vi "magazine_periodic.vi"(9 "Reverse":bool, 10 "Outtake":bool, 11 "Intake":bool) -> (2 "Stator Current":dbl)   [LabVIEW 2020]
uses:
  <vilib>/Rock Robotics/WPI/ThirdParty/Phoenix-LabVIEW/Motor Controller/Controls/CTRE_Phoenix_MotorControl_StatorCurrentLimitConfiguration.ctl
  <vilib>/Rock Robotics/WPI/ThirdParty/Phoenix-LabVIEW/Motor Controller/Controls/CTRE_Phoenix_MotorControl_ControlMode.ctl
  TitanLib/Lib/Piston Hold.vi
  <vilib>/Rock Robotics/WPI/Solenoid/WPI_SolenoidSetEnum.vi
  <vilib>/Rock Robotics/WPI/ThirdParty/Phoenix-LabVIEW/Motor Controller/Get/CTRE_Phoenix_MotorController_GetSupplyAndStatorCurrent_Enhanced.vi
  TitanLib/Lib/TitanLib.lvlib
panel:
  in  "Input":bool
  in  "Stator Current Limit Configuration":T1
  out "Sensor Values":cluster{i16, i16}(graph)
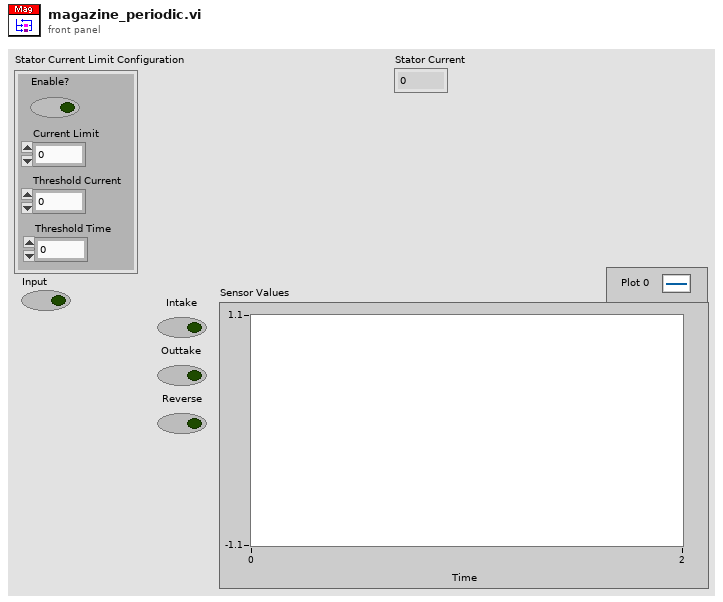
[diagram p1: front panel]
types:
  T1 = typedef "CTRE_Phoenix_MotorControl_StatorCurrentLimitConfiguration.ctl" = cluster{"Enable?":bool, "Current Limit":dbl, "Threshold Current":dbl, "Threshold Time":dbl}
  T2 = typedef "WPI_DigitalInputDevRef.ctl" = cluster{"DevStatus":errorcluster, "DIO Channel":T3}
  T3 = typedef "FPGA_DIOChannel.ctl" = enum8{"DIO 0", "DIO 1", "DIO 2", "DIO 3", "DIO 4", "DIO 5", "DIO 6", "DIO 7", "DIO 8", "DIO 9", "DIO MXP 0", "DIO MXP 1", "DIO MXP 2", "DIO MXP 3", "DIO MXP 4", "DIO MXP 5", "DIO MXP 6", "DIO MXP 7", "DIO MXP 8", "DIO MXP 9", "DIO MXP 10", "DIO MXP 11", "DIO MXP 12", "DIO MXP 13", "DIO MXP 14", "DIO MXP 15", "SPI Port CS1", "SPI Port CS2", "SPI Port CS3", "SPI Port MISO", "SPI Port MOSI", "Invalid"}
  T4 = typedef "WPI_SolenoidValue.ctl" = enum16{"Off", "On", "Forward", "Reverse"}
  T5 = typedef "WPI_SolenoidDevRef.ctl" = cluster{"DevStatus":errorcluster, "Pneumatics Control Module":u8, "Forward Solenoid Channel":T6, "Reverse Solenoid Channel":T6}
  T6 = typedef "WPI_SolenoidChannel.ctl" = enum8{"Solenoid 0", "Solenoid 1", "Solenoid 2", "Solenoid 3", "Solenoid 4", "Solenoid 5", "Solenoid 6", "Solenoid 7", "Solenoid 8", "Solenoid 9", "Solenoid 10", "Solenoid 11", "Solenoid 12", "Solenoid 13", "Solenoid 14", "Solenoid 15", "Invalid"}
  T7 = typedef "CTRE_Phoenix_MotorControl_ControlMode.ctl" = u16
  T8 = typedef "WPI_MotorControlDeviceRef.ctl" = cluster{"DeviceStatus":errorcluster, "Type":T9, "PWM":cluster{"PWM Channel":T10, "DeadBand":T11}, "CAN":cluster{"Device Number":u8, "SetOutput VI Ref":variant, "GetOutput VI Ref":variant, "Enable VI Ref":variant, "Disable VI Ref":variant, "Data":variant}, "Invert":bool, "DIO PWM":cluster{"PWM \"Enable\" Channel":T10, "DIOChannel":T3, "PWM Rate":dbl}}
  T9 = typedef "WPI_MotorControlType.ctl" = enum16{"PWM", "CAN", "DIO PWM"}
  T10 = typedef "FPGA_DIOPWMChannel.ctl" = enum8{"PWM 0", "PWM 1", "PWM 2", "PWM 3", "PWM 4", "PWM 5", "PWM 6", "PWM 7", "PWM 8", "PWM 9", "PWM MXP 0", "PWM MXP 1", "PWM MXP 2", "PWM MXP 3", "PWM MXP 4", "PWM MXP 5", "PWM MXP 6", "PWM MXP 7", "PWM MXP 8", "PWM MXP 9", "Invalid"}
  T11 = typedef "WPI_PWMDeadband.ctl" = cluster{"Name":string, "maxPositivePwm":i32, "minPositivePwm":i32, "centerPwm":i32, "maxNegativePwm":i32, "minNegativePwm":i32, "angularRange":u16}
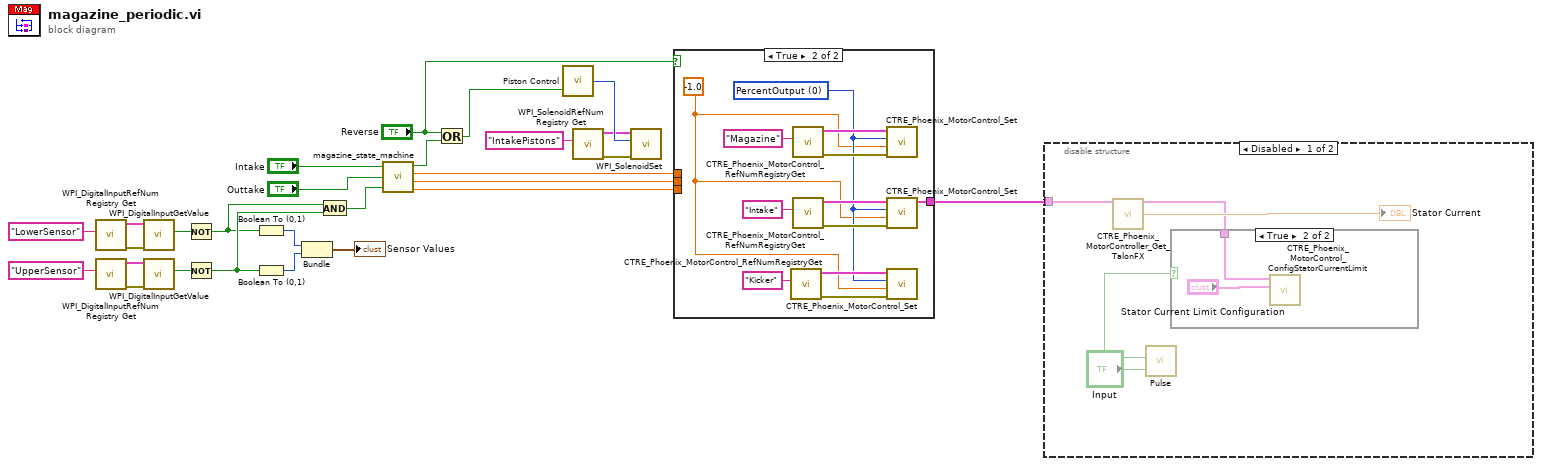
[diagram p0: block diagram]
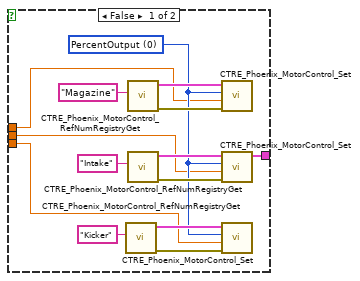
[diagram p4: hidden frame]
diagram:
  n1 = call <vilib>:"WPI_DigitalInputRefNum Registry Get.vi"("refnum name"="LowerSensor") -> ("error out"=w15:errorcluster, "DigitalInputDevRef"=w16:T2)  [unwired: 9 in]
  n2 = call <vilib>:"WPI_DigitalInputRefNum Registry Get.vi"("refnum name"="UpperSensor") -> ("error out"=w12:errorcluster, "DigitalInputDevRef"=w11:T2)  [unwired: 9 in]
  n3 = call <vilib>:"WPI_DigitalInputGetValue.vi"("error in (no error)"=w15, "DigitalInputDevRef"=w16) -> ("Value"=w19:bool)  [unwired: 7 in, 2 out]
  n4 = call <vilib>:"WPI_DigitalInputGetValue.vi"("error in (no error)"=w12, "DigitalInputDevRef"=w11) -> ("Value"=w20:bool)  [unwired: 7 in, 2 out]
  n5 = Not(x=w19) -> (.not. x?=w17:bool)
  n6 = Not(x=w20) -> (.not. x?=w18:bool)
  n7 = Boolean To (0,1)(Boolean=w17) -> (0, 1=w8:i16)
  n8 = Boolean To (0,1)(Boolean=w18) -> (0, 1=w9:i16)
  n9 = Bundle(w8, w9) -> (→"Sensor Values":cluster{i16, i16})  [unwired: 1 in]
  n10 = And(x=w17, y=w18) -> (x .and. y?=w21:bool)
  n11 = call "magazine_state_machine.vi"("Intake Button"="Intake", "Outtake Button"="Outtake", "Both Sensors Active?"=w21) -> ("Intake Pistons"=w25:bool, "Magazine Motor"=w26:dbl, "Intake Motor"=w23:dbl, "Kicker Motor"=w24:dbl)
  n12 = Or(x="Reverse", y=w25) -> (x .or. y?=w7:bool)
  n13 = call-poly "Piston Control.vi"("Input"=w7) -> ("Output"=w6:T4)  [unwired: 1 in]
  n14 = call <vilib>:"WPI_SolenoidRefNum Registry Get.vi"("refnum name"="IntakePistons") -> ("error out"=w3:errorcluster, "SolenoidDevRef"=w4:T5)  [unwired: 9 in]
  n15 = call-poly <vilib>:"WPI_SolenoidSet.vi"("error in (no error)"=w3, "Value"=w6, "SolenoidDevRef"=w4) -> ()  [unwired: 7 in, 2 out]
  n16 = case shown="True" "Reverse" {
    tunnel: w23 -> [w31 _]
    tunnel: w24 -> [w30 _]
    tunnel: w26 -> [w29 _]
    tunnel: [w28 w42] -> w1
    frame False {
      w32 = T7 0 items=["PercentOutput"=0, "Position"=1, "Velocity"=2, "Current"=3, "Follower"=5, "MotionProfile"=6, "MotionMagic"=7, "MotionProfileArc"=10, "Disabled"=15] ("Control Mode")
      n17 = call <vilib>:"CTRE_Phoenix_MotorControl_RefNumRegistryGet.vi"("refnum name"="Kicker") -> ("error out"=w39:errorcluster, "PhoenixMotorControlDevRef"=w38:T8)  [unwired: 9 in]
      n18 = call <vilib>:"CTRE_Phoenix_MotorControl_RefNumRegistryGet.vi"("refnum name"="Magazine") -> ("error out"=w41:errorcluster, "PhoenixMotorControlDevRef"=w40:T8)  [unwired: 9 in]
      n19 = call <vilib>:"CTRE_Phoenix_MotorControl_RefNumRegistryGet.vi"("refnum name"="Intake") -> ("error out"=w36:errorcluster, "PhoenixMotorControlDevRef"=w37:T8)  [unwired: 9 in]
      n20 = call <vilib>:"CTRE_Phoenix_MotorControl_Set.vi"("error in (no error)"=w41, "Output"=w29, "Control Mode"=w32, "PhoenixMotorControlDevRef"=w40) -> ()  [unwired: 6 in, 2 out]
      n21 = call <vilib>:"CTRE_Phoenix_MotorControl_Set.vi"("error in (no error)"=w36, "Output"=w31, "Control Mode"=w32, "PhoenixMotorControlDevRef"=w37) -> ("PhoenixMotorControlDevRef"=w28:T8)  [unwired: 6 in, 1 out]
      n22 = call <vilib>:"CTRE_Phoenix_MotorControl_Set.vi"("error in (no error)"=w39, "Output"=w30, "Control Mode"=w32, "PhoenixMotorControlDevRef"=w38) -> ()  [unwired: 6 in, 2 out]
    }
    frame True {
      w43 = -1.0 ("Output")
      w44 = T7 0 items=["PercentOutput"=0, "Position"=1, "Velocity"=2, "Current"=3, "Follower"=5, "MotionProfile"=6, "MotionMagic"=7, "MotionProfileArc"=10, "Disabled"=15] ("Control Mode")
      n23 = call <vilib>:"CTRE_Phoenix_MotorControl_RefNumRegistryGet.vi"("refnum name"="Kicker") -> ("error out"=w51:errorcluster, "PhoenixMotorControlDevRef"=w50:T8)  [unwired: 9 in]
      n24 = call <vilib>:"CTRE_Phoenix_MotorControl_RefNumRegistryGet.vi"("refnum name"="Magazine") -> ("error out"=w53:errorcluster, "PhoenixMotorControlDevRef"=w52:T8)  [unwired: 9 in]
      n25 = call <vilib>:"CTRE_Phoenix_MotorControl_RefNumRegistryGet.vi"("refnum name"="Intake") -> ("error out"=w48:errorcluster, "PhoenixMotorControlDevRef"=w49:T8)  [unwired: 9 in]
      n26 = call <vilib>:"CTRE_Phoenix_MotorControl_Set.vi"("error in (no error)"=w53, "Output"=w43, "Control Mode"=w44, "PhoenixMotorControlDevRef"=w52) -> ()  [unwired: 6 in, 2 out]
      n27 = call <vilib>:"CTRE_Phoenix_MotorControl_Set.vi"("error in (no error)"=w48, "Output"=w43, "Control Mode"=w44, "PhoenixMotorControlDevRef"=w49) -> ("PhoenixMotorControlDevRef"=w42:T8)  [unwired: 6 in, 1 out]
      n28 = call <vilib>:"CTRE_Phoenix_MotorControl_Set.vi"("error in (no error)"=w51, "Output"=w43, "Control Mode"=w44, "PhoenixMotorControlDevRef"=w50) -> ()  [unwired: 6 in, 2 out]
    }
  }
  n29 = disable-structure shown="Disabled" {
    disable-tunnel: w1 -> [w58 _]
    frame Disabled {
      n30 = call-poly <vilib>:"CTRE_Phoenix_MotorController_Get_TalonFX.vi"("PhoenixMotorControlDevRef"=w58) -> ("PhoenixMotorControlDevRef"=w56:T8, "Stator Current"=→"Stator Current":dbl)  [unwired: 11 in, 2 out]
      n31 = call "Pulse.vi"("Input"="Input") -> ("Output"=w55:bool)  [unwired: 10 in]
      n32 = case shown="True" w55 {
        tunnel: w56 -> [_ w60]
        frame False {
        }
        frame True {
          n33 = call <vilib>:"CTRE_Phoenix_MotorControl_ConfigStatorCurrentLimit.vi"("Stator Current Limit Configuration"="Stator Current Limit Configuration", "PhoenixMotorControlDevRef"=w60) -> ()  [unwired: 8 in, 2 out]
        }
      }
    }
    frame Enabled {
    }
  }
